vi "PS35_CmdAns.vi"(4 "error in (no error)":errorcluster, 5 "nRequest":i32 min=0 max=1, 6 "Command":string, 7 "Control unit ID":i32=1 min=1 max=10) -> (0 "error out":errorcluster, 1 "String length":i32, 2 "Answer string":string)   [LabVIEW 2020]
doc: "PS35_CmdAns.vi, created: 06.03.2009 alex; last change: 22.10.2019 alex;\n\n<B>FUNCTION:</B> \n\nSend direct commands to the control unit (low level communication).\nOne can communicate with this function with the control unit directly. \nThe commands from the command reference of the control unit are used.\nThe maximum size of the communication buffer is 100 characters.\n----------------------------------------------------------------------------------------\n<B>INPUT:</B>\n[I32] <B>Control unit ID:</B> control unit index. (Default=1, Range=1...10)\n[CStr] <B>Command:</B> command from the command reference. (Default=empty string) \n[I32] <B>nRequest:</B> request mode. (Default=0, Range=0...1)\n0 - send command to the control unit (no request),\n1 - send command and after that read answer.\n[CLU] <B>error in</B>\n----------------------------------------------------------------------------------------\n<B>OUTPUT:</B>\n[CStr] <B>Answer string:</B> answer from the control unit.\n[I32] <B>String length:</B> length of the answer string.\n[CLU] <B>error out</B>\n----------------------------------------------------------------------------------------\n<B>SUB-VIs:</B>\nPS35_GetReadError.vi\n----------------------------------------------------------------------------------------\n<B>EXT-Calls:</B>\nps35.dll (V2.01)\n----------------------------------------------------------------------------------------"
uses:
  ps35.dll
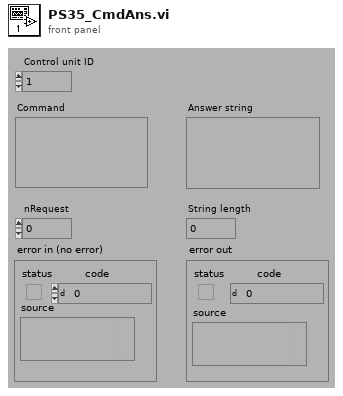
[diagram p1: front panel]
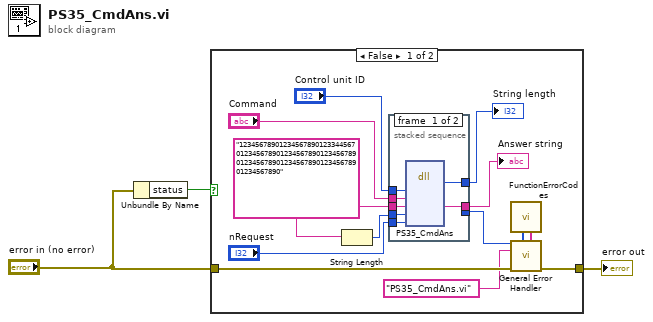
[diagram p0: block diagram]
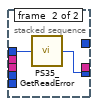
[diagram p2: hidden frame]
diagram:
  n1 = Unbundle By Name("error in (no error)") -> ("status"=w1:bool)
  n2 = case shown="False" w1 {
    tunnel: "error in (no error)" -> [w15 w26]
    tunnel: [w14 w26] -> w3
    frame False {
      w9 = "1234567890123456789012334456701234567890123456789012345678901234567890123456789012345678901234567890"
      n3 = String Length(string=w9) -> (length=w10:i32)
      n4 = stacked-sequence {
        tunnel: "Control unit ID" -> [w23 w25]
        tunnel: [w22 _] -> w13
        tunnel: [_ w24] -> w12
        tunnel: [w21 _] -> w11
        tunnel: w10 -> [w20 _]
        tunnel: w9 -> [w19 _]
        tunnel: "Command" -> [w18 _]
        tunnel: "nRequest" -> [w17 _]
        frame #0 {
          n5 = dll-call lib="C:/GEECS/Developers Version/source/Device Drivers/OwiSoft/OWISoftOEM/ps35/labview/lv82/ps35.dll" fn="PS35_CmdAns" label="PS35_\nCmdAns"("Index"=w23, "szCmd"=w18, "szAns"=w19, "Length"=w20, "nRequest"=w17) -> ("Rückgabetyp"=w22:i32, "szAns"=w21:string)  [unwired: 7 in, 2 out]
        }
        frame #1 {
          n6 = call "PS35_GetReadError.vi"("Control unit ID"=w25) -> ("Read error"=w24:i32)
        }
      }
      "Answer string" <- w11
      "String length" <- w13
      n7 = call "FunctionErrorCodes.vi"() -> ("[user-defined codes]"=w5:i32[], "[user-defined descriptions]"=w4:string[])  [unwired: 8 in]
      n8 = call <vilib>:"General Error Handler.vi"("[error code] (0)"=w12, "[user-defined codes]"=w5, "[user-defined descriptions]"=w4, "[error source] (\" \")"="PS35_CmdAns.vi" ("[error source] (\" \")"), "error in (no error)"=w15) -> ("error out"=w14:errorcluster)  [unwired: 6 in, 4 out]
    }
    frame True {
    }
  }
  "error out" <- w3
